vi "Periodic Tasks.vi"(8 "error in":errorcluster) -> ()   [LabVIEW 2019]
doc: "This VI runs in parallel to other tasks. It can contain as many user-defined periodic loops as you need. These can carry out PID or other sorts of timed response."
uses:
  <vilib>/Rock Robotics/WPI/Utilities/WPI_GetSetVariantRefNum.vi
  <vilib>/Rock Robotics/WPI/Ultrasonic/WPI_SonarSRF04DigitalRefNum Registry Get.vi
  <vilib>/Rock Robotics/Network Tables/NT Read Number.vi
  Robot Global Data.vi
  <vilib>/Rock Robotics/Network Tables/NT Write Number.vi
  <vilib>/Rock Robotics/WPI/Ultrasonic/WPI_SonarSRF04DigitalGetRange.vi
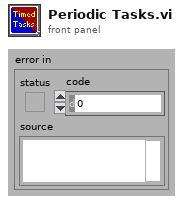
[diagram p1: front panel]
types:
  T1 = typedef "WPI_JoystickDevRef.ctl" = cluster{"Device":T2}
  T2 = typedef "WPI_JoystickDeviceEnum.ctl" = enum16{"USB 0", "USB 1", "USB 2", "USB 3", "USB 4", "USB 5"}
  T3 = typedef "WPI_RobotDriveDevRef.ctl" = cluster{"DevStatus":errorcluster, "Motors[]":T4[], "Square Inputs":bool, "Max Output":dbl}
  T4 = typedef "WPI_MotorControlDeviceRef.ctl" = cluster{"DeviceStatus":errorcluster, "Type":T5, "PWM":cluster{"PWM Channel":T6, "DeadBand":T7}, "CAN":cluster{"Device Number":u8, "SetOutput VI Ref":variant, "GetOutput VI Ref":variant, "Enable VI Ref":variant, "Disable VI Ref":variant, "Data":variant}, "Invert":bool, "DIO PWM":cluster{"PWM \"Enable\" Channel":T6, "DIOChannel":T8, "PWM Rate":dbl}}
  T5 = typedef "WPI_MotorControlType.ctl" = enum16{"PWM", "CAN", "DIO PWM"}
  T6 = typedef "FPGA_DIOPWMChannel.ctl" = enum8{"PWM 0", "PWM 1", "PWM 2", "PWM 3", "PWM 4", "PWM 5", "PWM 6", "PWM 7", "PWM 8", "PWM 9", "PWM MXP 0", "PWM MXP 1", "PWM MXP 2", "PWM MXP 3", "PWM MXP 4", "PWM MXP 5", "PWM MXP 6", "PWM MXP 7", "PWM MXP 8", "PWM MXP 9", "Invalid"}
  T7 = typedef "WPI_PWMDeadband.ctl" = cluster{"Name":string, "maxPositivePwm":i32, "minPositivePwm":i32, "centerPwm":i32, "maxNegativePwm":i32, "minNegativePwm":i32, "angularRange":u16}
  T8 = typedef "FPGA_DIOChannel.ctl" = enum8{"DIO 0", "DIO 1", "DIO 2", "DIO 3", "DIO 4", "DIO 5", "DIO 6", "DIO 7", "DIO 8", "DIO 9", "DIO MXP 0", "DIO MXP 1", "DIO MXP 2", "DIO MXP 3", "DIO MXP 4", "DIO MXP 5", "DIO MXP 6", "DIO MXP 7", "DIO MXP 8", "DIO MXP 9", "DIO MXP 10", "DIO MXP 11", "DIO MXP 12", "DIO MXP 13", "DIO MXP 14", "DIO MXP 15", "SPI Port CS1", "SPI Port CS2", "SPI Port CS3", "SPI Port MISO", "SPI Port MOSI", "Invalid"}
  T9 = typedef "WPI_UltrasonicDeviceRef.ctl" = cluster{"DevStatus":errorcluster, "Ping Channel":T8, "Echo Channel":T8, "CntIndex":T10}
  T10 = typedef "FPGA_CounterCtrSystemIndex.ctl" = enum8{"Ctr 0", "Ctr 1", "Ctr 2", "Ctr 3", "Ctr 4", "Ctr 5", "Ctr 6", "Ctr 7", "Invalid"}
  T11 = typedef "WPI_GyroDevRef.ctl" = cluster{"DevStatus":errorcluster, "Analog Channel":T12, "Gain (VoltsPerDegree/Second)":dbl, "Gyro Type":enum16{"Analog", "XRS450"}, "Handle":i32, "SPI Bus":T13, "Device Found":bool, "Sample Rate":dbl, "Calibrate On Open":bool, "Offset":dbl}
  T12 = typedef "FPGA_AIChannel.ctl" = enum8{"AI 0", "AI 1", "AI 2", "AI 3", "AI MXP 0", "AI MXP 1", "AI MXP 2", "AI MXP 3", "Invalid"}
  T13 = typedef "spi_bus.ctl" = enum16{"SPI On-Board, CS0", "SPI On-Board, CS1", "SPI On-Board, CS2", "SPI On-Board, CS3", "SPI MXP", "Invalid"}
  T14 = cluster{"JoystickDevRef":T1, "RobotDriveDevRef":T3}
  T15 = typedef "WPI_ServoDeviceRef.ctl" = cluster{"DeviceStatus":errorcluster, "PWM Channel":T6, "DeadBand":T7}
  T16 = typedef "WPI_DriverStationRobotMode2.ctl" = enum16{"Autonomous Disabled", "Autonomous Enabled", "Teleop Disabled", "Teleop Enabled", "Disconnected", "Finish", "Test Disabled", "Test Enabled", "Emergency Stopped"}
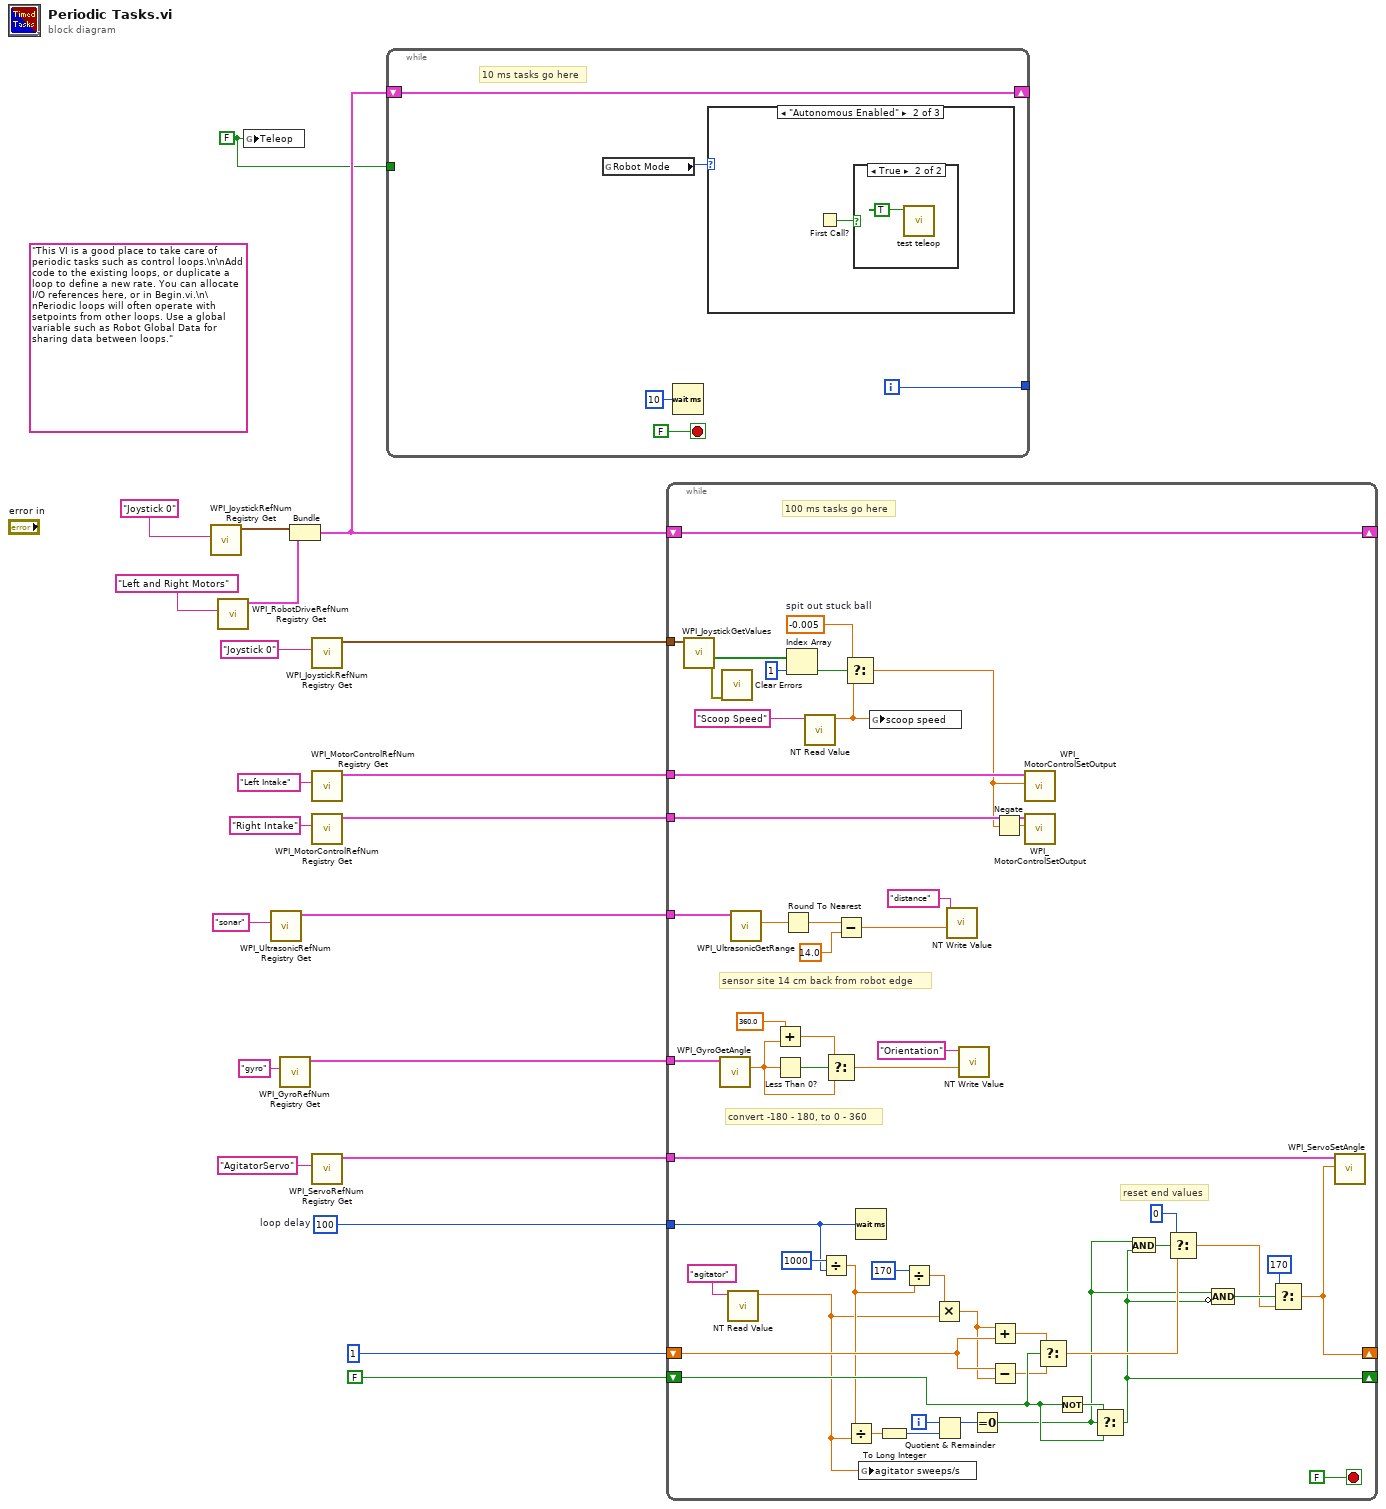
[diagram p0: block diagram]
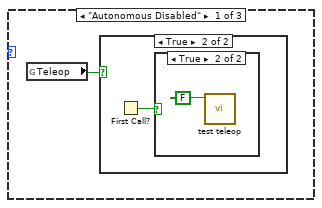
[diagram p2: hidden frame]
diagram:
  w1 = FALSE ("Teleop")
  w6 = u32 100  # loop delay
  (unwired) "This VI is a good place to take care of periodic tasks such as control loops.\n\nAdd code to the existing loops, or duplicate a loop to define a new rate. You can allocate I/O references here, or in Begin.vi.\n\nPeriodic loops will often operate with setpoints from other loops. Use a global variable such as Robot Global Data for sharing data between loops."
  n1 = call <vilib>:"WPI_JoystickRefNum Registry Get.vi"("refnum name"="Joystick 0") -> ("JoystickDevRef"=w19:T1)  [unwired: 1 in, 9 out]
  n2 = call <vilib>:"WPI_RobotDriveRefNum Registry Get.vi"("refnum name"="Left and Right Motors") -> ("RobotDriveDevRef"=w18:T3)  [unwired: 1 in, 9 out]
  n3 = global write "Robot Global Data.vi" "Teleop"(w1) -> ()
  n4 = call-poly <vilib>:"WPI_UltrasonicRefNum Registry Get.vi"("refnum name"="sonar") -> ("SonarSRF04DevRef"=w4:T9)  [unwired: 9 in, 1 out]
  n5 = call <vilib>:"WPI_GyroRefNum Registry Get.vi"("refnum name"="gyro") -> ("GyroDevRef"=w2:T11)  [unwired: 9 in, 1 out]
  n6 = Bundle("JoystickDevRef"=w19, "RobotDriveDevRef"=w18) -> (w17:T14)  [unwired: 1 out]
  n7 = call <vilib>:"WPI_JoystickRefNum Registry Get.vi"("refnum name"="Joystick 0") -> ("JoystickDevRef"=w7:T1)  [unwired: 1 in, 9 out]
  n8 = call <vilib>:"WPI_MotorControlRefNum Registry Get.vi"("refnum name"="Left Intake") -> ("MotorControlDevRef"=w12:T4)  [unwired: 9 in, 1 out]
  n9 = call <vilib>:"WPI_MotorControlRefNum Registry Get.vi"("refnum name"="Right Intake") -> ("MotorControlDevRef"=w9:T4)  [unwired: 9 in, 1 out]
  n10 = call <vilib>:"WPI_ServoRefNum Registry Get.vi"("refnum name"="AgitatorServo") -> ("ServoDeviceRef"=w15:T15)  [unwired: 9 in, 1 out]
  n11 = while {
    shift-right: [w24] -> _
    shift-left: w17 -> [w24]
    tunnel: [w22] -> _
    tunnel: w1 -> [_]
    i -> [w22]
    stop <- FALSE stop-if-true
    # "10 ms tasks go here"
    n12 = global read "Robot Global Data.vi" "Robot Mode"() -> (w23:T16)
    n13 = Wait (ms)(milliseconds to wait=u32 10) -> ()  [unwired: 1 out]
    n14 = case shown="\"Autonomous Enabled\"" w23 {
      frame "Autonomous Disabled" {
        n15 = global read "Robot Global Data.vi" "Teleop"() -> (w27:bool)
        n16 = case shown="True" w27 {
          frame False {
          }
          frame True {
            n17 = First Call?() -> (First Call?: T/F=w28:bool)
            n18 = case shown="True" w28 {
              frame False {
              }
              frame True {
                n19 = call "test teleop.vi"("Boolean"=FALSE) -> ()  [unwired: 10 in, 1 out]
              }
            }
          }
        }
      }
      frame "Autonomous Enabled" {
        n20 = First Call?() -> (First Call?: T/F=w30:bool)
        n21 = case shown="True" w30 {
          frame False {
          }
          frame True {
            n22 = call "test teleop.vi"("Boolean"=TRUE) -> ()  [unwired: 10 in, 1 out]
          }
        }
      }
      frame "Teleop Disabled", Default {
      }
    }
  }
  n23 = while {
    shift-right: [w84] -> _
    shift-left: w17 -> [w84]
    tunnel: w15 -> [w83]
    shift-right: [w51] -> _
    shift-left: 1 ("Angle") -> [w65]
    shift-right: [w54] -> _
    shift-left: FALSE -> [w70]
    tunnel: w12 -> [w79]
    tunnel: w9 -> [w78]
    tunnel: w7 -> [w76]
    tunnel: w6 -> [w67]
    tunnel: w4 -> [w47]
    tunnel: w2 -> [w41]
    i -> [w82]
    stop <- FALSE stop-if-true
    w71 = -0.005  # spit out stuck ball
    # "convert -180 - 180, to 0 - 360"
    # "sensor site 14 cm back from robot edge"
    # "reset end values"
    # "100 ms tasks go here"
    n24 = call <vilib>:"WPI_JoystickGetValues.vi"("JoystickDevRef"=w76) -> ("error out"=w32:errorcluster, "Buttons"=w75:bool[])  [unwired: 6 in, 3 out]
    n25 = call <vilib>:"WPI_GyroGetAngle.vi"("GyroDevRef"=w41) -> ("Angle"=w36:dbl)  [unwired: 7 in, 3 out]
    n26 = call <vilib>:"Clear Errors.vi"("error in (no error)"=w32) -> ()  [unwired: 5 in, 2 out]
    n27 = call-poly <vilib>:"NT Read Value.vi"("Name"="agitator") -> ("Numeric"=w33:dbl)  [unwired: 9 in, 1 out]
    n28 = call-poly <vilib>:"WPI_UltrasonicGetRange.vi"("UltrasonicDevRef"=w47) -> ("Distance"=w46:dbl)  [unwired: 8 in, 2 out]
    n29 = Add(x=360.0, y=w36) -> (x+y=w37:dbl)
    n30 = Less Than 0?(x=w36) -> (x < 0?=w39:bool)
    n31 = Round To Nearest(number=w46) -> (nearest integer value=w44:dbl)
    n32 = Index Array(array=w75, index=1) -> (element=w73:bool)
    n33 = call-poly <vilib>:"NT Read Value.vi"("Name"="Scoop Speed") -> ("Numeric"=w48:dbl)  [unwired: 9 in, 1 out]
    n34 = Divide(x=u32 1000 ("loop delay"), y=w67) -> (x/y=w63:dbl)
    n35 = Select(t=w37, s=w39, f=w36) -> (s? t:f=w38:dbl)
    n36 = Subtract(x=w44, y=14.0) -> (x-y=w43:dbl)
    n37 = Select(t=w71, s=w73, f=w48) -> (s? t:f=w72:dbl)
    n38 = Divide(x=w63, y=w33) -> (x/y=w61:dbl)
    n39 = Wait (ms)(milliseconds to wait=w67) -> ()  [unwired: 1 out]
    n40 = global write "Robot Global Data.vi" "agitator sweeps/s"(w33) -> ()
    n41 = global write "Robot Global Data.vi" "scoop speed"(w48) -> ()
    n42 = To Long Integer(number=w61) -> (32bit integer=w59:i32)
    n43 = Divide(x=170 ("y"), y=w63) -> (x/y=w62:dbl)
    n44 = Multiply(x=w62, y=w33) -> (x*y=w60:dbl)
    n45 = Quotient & Remainder(x=w82, y=w59) -> (x-y*floor(x/y)=w81:i32)  [unwired: 1 out]
    n46 = call-poly <vilib>:"NT Write Value.vi"("Numeric"=w43, "Name"="distance") -> ()  [unwired: 9 in, 1 out]
    n47 = call-poly <vilib>:"NT Write Value.vi"("Numeric"=w38, "Name"="Orientation") -> ()  [unwired: 9 in, 1 out]
    n48 = Equal To 0?(x=w81) -> (x = 0?=w55:bool)
    n49 = Add(x=w60, y=w65) -> (x+y=w66:dbl)
    n50 = Subtract(x=w65, y=w60) -> (x-y=w69:dbl)
    n51 = Negate(x=w72) -> (-x=w77:dbl)
    n52 = call <vilib>:"WPI_MotorControlSetOutput.vi"("Output"=w72, "MotorControlDevRef"=w79) -> ()  [unwired: 7 in, 3 out]
    n53 = call <vilib>:"WPI_MotorControlSetOutput.vi"("Output"=w77, "MotorControlDevRef"=w78) -> ()  [unwired: 7 in, 3 out]
    n54 = Select(t=w66, s=w70, f=w69) -> (s? t:f=w56:dbl)
    n55 = Not(x=w70) -> (.not. x?=w80:bool)
    n56 = Select(t=w80, s=w55, f=w70) -> (s? t:f=w54:bool)
    n57 = And(x=w55, y=w54) -> (x .and. y?=w58:bool)
    n58 = Select(t=0 ("y"), s=w58, f=w56) -> (s? t:f=w52:dbl)
    n59 = Compound Arithmetic op=AND(w55, invert w54) -> (w53:bool)
    n60 = Select(t=170 ("y"), s=w53, f=w52) -> (s? t:f=w51:dbl)
    n61 = call <vilib>:"WPI_ServoSetAngle.vi"("Angle"=w51, "ServoDeviceRef"=w83) -> ()  [unwired: 8 in, 2 out]
  }
